vi "KalmanCalculationAux.vi"(6 "R":T1, 9 "A + B in":T1, 10 "A + B 3":T1, 11 "z_k":T1) -> (2 "A - B":T1, 3 "A + B out":T1)   [LabVIEW 2018]
uses:
  <vilib>/Analysis/Matrix/Datatypes/RealMatrix.ctl
  <vilib>/Analysis/Matrix/Numeric/Multiply/Multiply - RM,RM.vi
  <vilib>/Analysis/Matrix/Numeric/Subtract/Subtract - RM,RM.vi
  <vilib>/Analysis/Matrix/Numeric/Add/Add - RM,RM.vi
  <vilib>/Analysis/baseanly.llb/Real Inverse Matrix.vi
  <vilib>/Analysis/Matrix/NI_Matrix.lvlib
  <vilib>/Analysis/NI_AALBase.lvlib
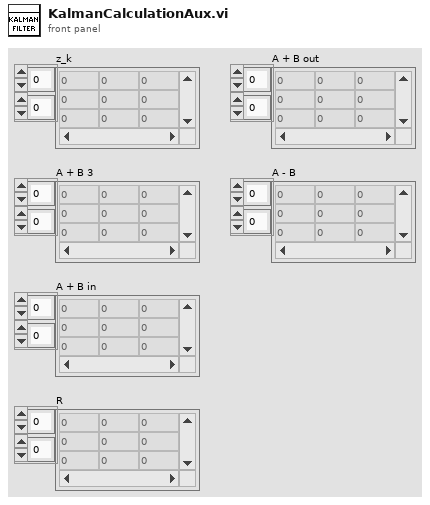
[diagram p1: front panel]
types:
  T1 = typedef "NI_Matrix.lvlib/RealMatrix.ctl" = dbl[][]
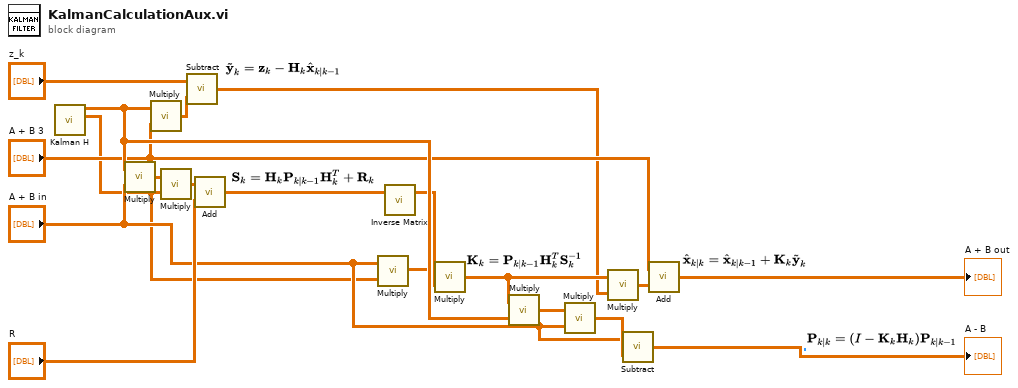
[diagram p0: block diagram]
diagram:
  n1 = call "Kalman H.vi"() -> ("H'"=w6:T1, "H"=w13:T1)  [unwired: 10 in]
  n2 = call-poly <vilib>:"Multiply.vi"("Real Matrix B"="A + B in", "Real Matrix A"=w13) -> ("A * B"=w3:T1)
  n3 = call-poly <vilib>:"Multiply.vi"("Real Matrix B"="A + B 3", "Real Matrix A"=w13) -> ("A * B"=w2:T1)
  n4 = call-poly <vilib>:"Multiply.vi"("Real Matrix B"=w6, "Real Matrix A"=w3) -> ("A * B"=w4:T1)
  n5 = call-poly <vilib>:"Subtract.vi"("Real Matrix B"=w2, "Real Matrix A"="z_k") -> ("A - B"=w9:T1)
  n6 = call-poly <vilib>:"Add.vi"("Real Matrix B"="R", "Real Matrix A"=w4) -> ("A + B"=w5:T1)
  n7 = call-poly <vilib>:"Multiply.vi"("Real Matrix B"=w6, "Real Matrix A"="A + B in") -> ("A * B"=w7:T1)
  n8 = call-poly <vilib>:"Inverse Matrix.vi"("Input Matrix"=w5) -> ("Inverse Matrix"=w8:T1)  [unwired: 1 in, 1 out]
  n9 = call-poly <vilib>:"Multiply.vi"("Real Matrix B"=w8, "Real Matrix A"=w7) -> ("A * B"=w12:T1)
  n10 = call-poly <vilib>:"Multiply.vi"("Real Matrix B"=w13, "Real Matrix A"=w12) -> ("A * B"=w14:T1)
  n11 = call-poly <vilib>:"Multiply.vi"("Real Matrix B"="A + B in", "Real Matrix A"=w14) -> ("A * B"=w16:T1)
  n12 = call-poly <vilib>:"Multiply.vi"("Real Matrix B"=w9, "Real Matrix A"=w12) -> ("A * B"=w10:T1)
  n13 = call-poly <vilib>:"Subtract.vi"("Real Matrix B"=w16, "Real Matrix A"="A + B in") -> ("A - B"=→"A - B":T1)
  n14 = call-poly <vilib>:"Add.vi"("Real Matrix B"=w10, "Real Matrix A"="A + B 3") -> ("A + B"=→"A + B out":T1)
